vi "myRIO_BRig_RT_dataCurrent_count_generic.vi"() -> (2 "output_count_generic":i32)   [LabVIEW 2014]
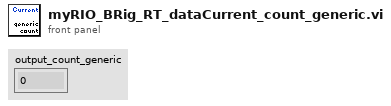
[diagram p1: front panel]
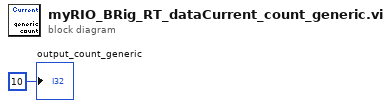
[diagram p0: block diagram]
diagram:
  "output_count_generic" <- 10 ("output_iBlock")
